vi "Clone Registration AE.vi"(0 "Module ID":i32=-1, 1 "Action":T1=enum."Add Instance", 11 "error in (no error)":errorcluster) -> (2 "empty":bool, 3 "Instances Names":string[](array[string]), 4 "Module IDs":i32[](array[numeric]), 6 "First Module ID":i32, 8 "replaced":bool, 10 "Found?":bool, 13 "First?":bool, 14 "First? (all)":bool[](array[boolean]), 15 "error out":errorcluster)   [LabVIEW 2014, in "GenNet-Client.lvlib" / "Clone Registration.lvlib"]
doc: "A registry (implemented as an Action Engine) to store all cloneable module instances. The Action Engine data is stored in a variant attribute table.\n\nOutput <b>First? </b> : We care which module instance was the first as the lifetime of the event references is bound to the lifetime of the module that created them (ie the first module instance). To avoid event references going bad we keep track of the first module and do not close it until safe to do so (ie when all other instances have closed).\n\nIf the first instance is closed whilst others are still running we effectively set that instance to idle. We deregister for all requests except STOP ALL.\n_____\nBased on Delacor QMH Project Template 3.1.0.34.\n\n<b>Note:</b> This VI was modified by the <b>Validate DQMH Module</b> tool to upgrade it to the DQMH 5.0 approach to destroying cloneable module event references."
uses:
  Clone Registration.lvlib
  Action--enum.ctl
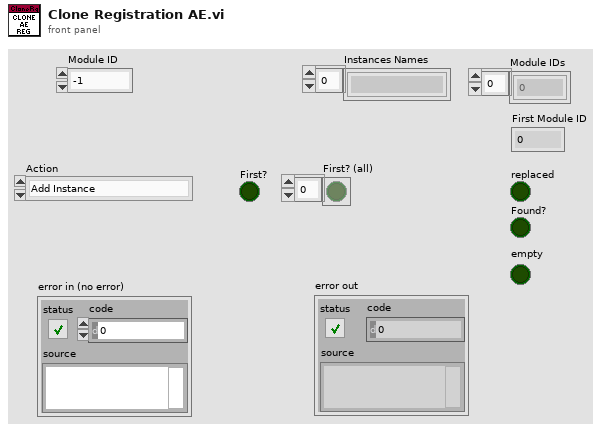
[diagram p1: front panel]
types:
  T1 = typedef "GenNet-Client.lvlib/Clone Registration.lvlib/Action--enum.ctl" = enum16{"Init", "Add Instance", "Remove Instance", "List Instances", "Is First?"}
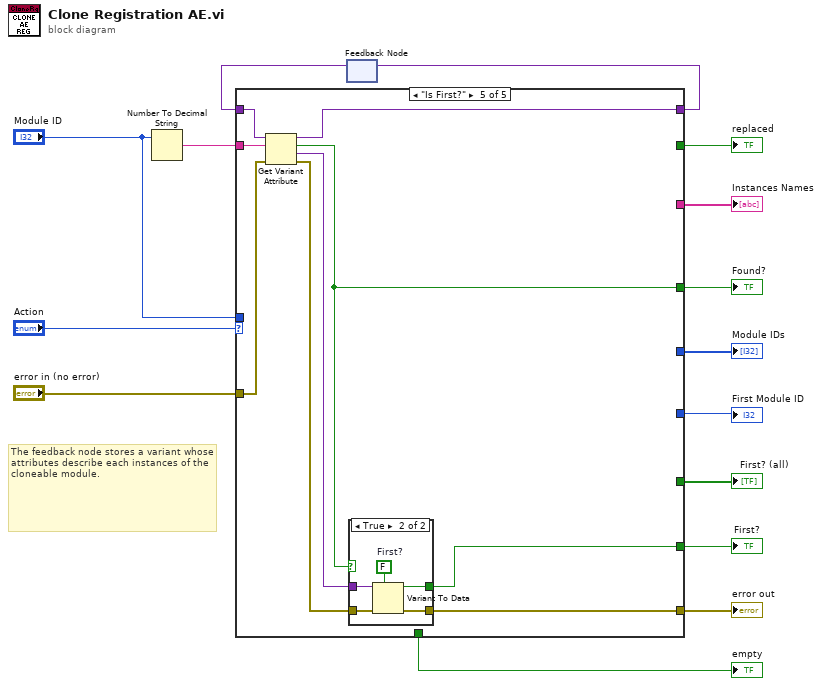
[diagram p0: block diagram]
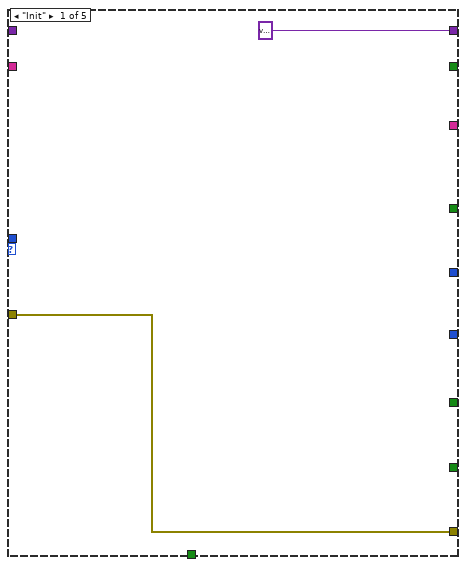
[diagram p2: hidden frame]
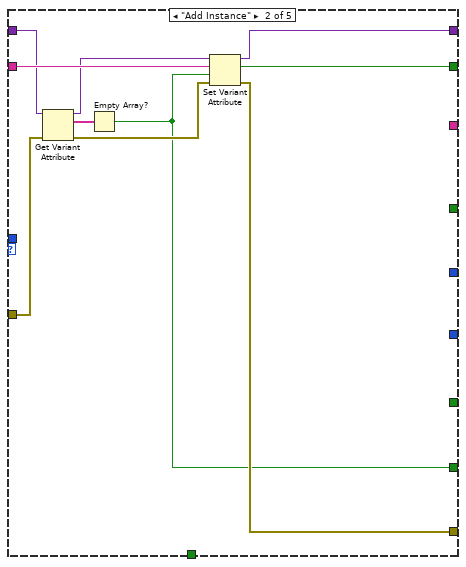
[diagram p3: hidden frame]
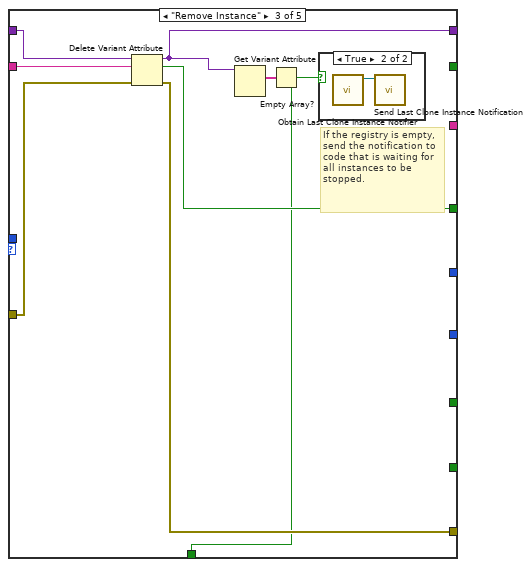
[diagram p4: hidden frame]
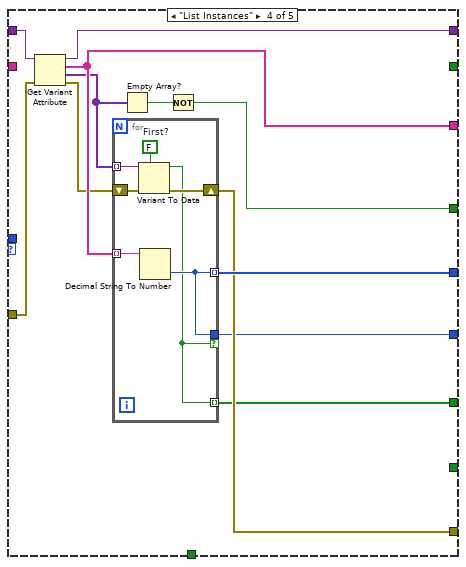
[diagram p6: hidden frame]
diagram:
  # "The feedback node stores a variant whose attributes describe each instances of the cloneable module."
  n1 = Number To Decimal String(number="Module ID") -> (decimal integer string=w14:string)  [unwired: 1 in]
  n2 = feedback #1() -> (w12:variant)  [unwired: 1 in]
  n3 = case shown="\"Is First?\"" "Action" {
    tunnel: w12 -> [_ w24 w35 w48 w64]
    tunnel: [variant w27 w34 w47 w63] -> w11
    tunnel: w14 -> [_ w26 w33 _ w58]
    tunnel: [_ w25 _ _ _] -> w10
    tunnel: [_ _ w32 w45 w56] -> w9
    tunnel: "Module ID" -> [_ _ _ _ _]
    tunnel: [_ _ _ w44 _] -> w8
    tunnel: [_ _ _ w43 _] -> w7
    tunnel: [_ _ _ w38 _] -> w6
    tunnel: "error in (no error)" -> [w16 w21 w31 w41 w61]
    tunnel: [w16 w19 w30 w39 w59] -> w4
    tunnel: [_ _ _ w37 _] -> w3
    tunnel: [_ w18 _ _ w57] -> w2
    tunnel: [_ _ w29 _ _] -> w1
    frame "Init" {
    }
    frame "Add Instance" {
      n4 = Get Variant Attribute(Variant=w24, error in=w21) -> (duplicate Variant=w23:variant, names=w22:string[], error out=w20:errorcluster)  [unwired: 2 in, 1 out]
      n5 = Empty Array?(array=w22) -> (empty?=w18:bool)
      n6 = Set Variant Attribute(Variant=w23, name=w26, value=w18, error in=w20) -> (Variant out=w27:variant, replaced=w25:bool, error out=w19:errorcluster)
    }
    frame "Remove Instance" {
      # "If the registry is empty, send the notification to code that is waiting for all instances to be stopped."
      n7 = Delete Variant Attribute(4:w31, 6:w33, 7:w35) -> (0:w30:errorcluster, 2:w32:bool, 3:w34:variant)
      n8 = Get Variant Attribute(Variant=w34) -> (names=w28:string[])  [unwired: 3 in, 3 out]
      n9 = Empty Array?(array=w28) -> (empty?=w29:bool)
      n10 = case shown="True" w29 {
        frame False {
        }
        frame True {
          n11 = call "Obtain Last Clone Instance Notifier.vi"() -> ("Last Instance Notifier"=w36:refnum<notifier>)  [unwired: 10 in, 1 out]
          n12 = call "Send Last Clone Instance Notification.vi"("Last Instance Notifier"=w36) -> ()  [unwired: 11 in]
        }
      }
    }
    frame "List Instances" {
      n13 = Get Variant Attribute(Variant=w48, error in=w41) -> (duplicate Variant=w47:variant, names=w43:string[], values=w42:variant[], error out=w40:errorcluster)  [unwired: 2 in]
      n14 = for {
        tunnel: w43 -> [w55] mode=indexing
        tunnel: [w50] -> w44 mode=indexing
        tunnel: w42 -> [w54] mode=indexing
        shift-right: [w51] -> w39
        shift-left: w40 -> [w52]
        tunnel: [w49] -> w38 mode=indexing
        tunnel: [w50] -> w37 if=w49
        w53 = FALSE  # First?
        n15 = Variant To Data(error in=w52, type=w53, Variant=w54) -> (data=w49:bool, error out=w51:errorcluster)
        n16 = Decimal String To Number(string=w55) -> (number=w50:i32)  [unwired: 2 in, 1 out]
      }
      n17 = Empty Array?(array=w42) -> (empty?=w46:bool)
      n18 = Not(x=w46) -> (.not. x?=w45:bool)
    }
    frame "Is First?" {
      n19 = Get Variant Attribute(Variant=w64, name=w58, error in=w61) -> (duplicate Variant=w63:variant, found=w56:bool, value=w62:variant, error out=w60:errorcluster)  [unwired: 1 in]
      n20 = case shown="True" w56 {
        tunnel: w62 -> [_ w70]
        tunnel: w60 -> [w65 w69]
        tunnel: [w65 w68] -> w59
        tunnel: [_ w66] -> w57
        frame False {
        }
        frame True {
          w67 = FALSE  # First?
          n21 = Variant To Data(error in=w69, type=w67, Variant=w70) -> (data=w66:bool, error out=w68:errorcluster)
        }
      }
    }
  }
  "replaced" <- w10
  "Found?" <- w9
  "Module IDs" <- w8
  "Instances Names" <- w7
  "First? (all)" <- w6
  "error out" <- w4
  "First Module ID" <- w3
  "First?" <- w2
  "empty" <- w1
  n22 = feedback-in #1(w11) -> ()
